vi "Actor Teardown Core.vi"(7 "Actor":refnum<class "Actor.lvclass">, 10 "Error":errorcluster, 11 "Destroying Self Actor State in":refnum<class "Destroying Self Actor State.lvclass">) -> (0 "error out":errorcluster, 2 "Teardown?":bool)   [LabVIEW 2021, in "jettl.lvlib" / "Destroying Self Actor State.lvclass"]
uses:
  Destroying Self Actor State.lvclass
  Actor/Actor.lvclass
  Msgs/Actor Last Ack/Actor Last Ack Msg Strategy/Actor Last Ack Msg Strategy.lvclass
  C:/git/jettl/src/LVCAM/LVCAM/Msg Strategy/Msg Strategy.lvclass
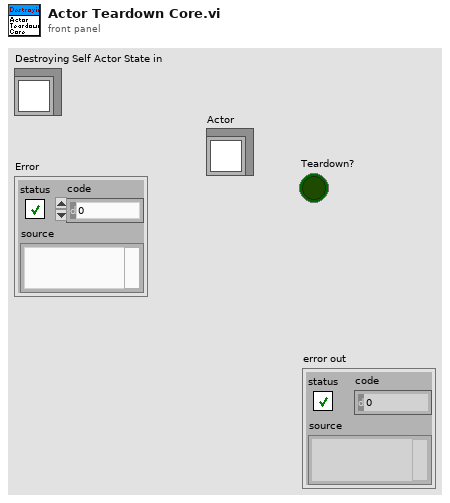
[diagram p1: front panel]
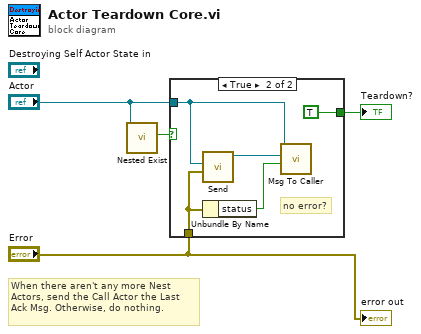
[diagram p0: block diagram]
diagram:
  # "When there aren't any more Nest Actors, send the Call Actor the Last Ack Msg. Otherwise, do nothing."
  n1 = call-dynamic "Nested Exist.vi"("Actor in"="Actor") -> ("Nested Exist?"=w3:bool)  [unwired: 10 in]
  n2 = case shown="True" w3 {
    tunnel: "Actor" -> [_ w7]
    tunnel: "Error" -> [_ w8]
    tunnel: [_ TRUE ("Destroyed?")] -> w4
    frame False {
    }
    frame True {
      # "no error?"
      n3 = call "Send.vi"("Nested Error"=w8, "Nested Actor"=w7) -> ("Actor Last Ack Msg Strategy out"=w6:refnum<class "Actor Last Ack Msg Strategy.lvclass">)  [unwired: 9 in]
      n4 = Unbundle By Name(w8) -> ("status"=w5:bool)
      n5 = call-dynamic "Msg To Caller.vi"("Priority Msg?"=w5, "Msg"=w6, "Actor in"=w7) -> ()  [unwired: 8 in, 1 out]
    }
  }
  "Teardown?" <- w4
  "error out" <- "Error"
